vi "newest map.vi"() -> (1 "newest map":path[](array[path]))   [LabVIEW 2014]
panel:
  out "last mod":timestamp
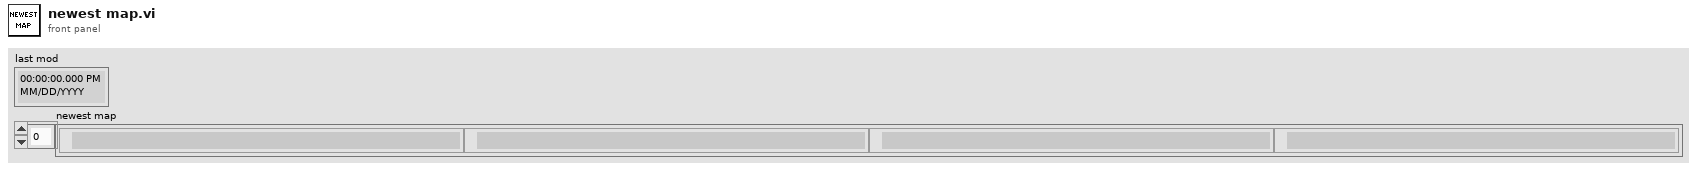
[diagram p1: front panel]
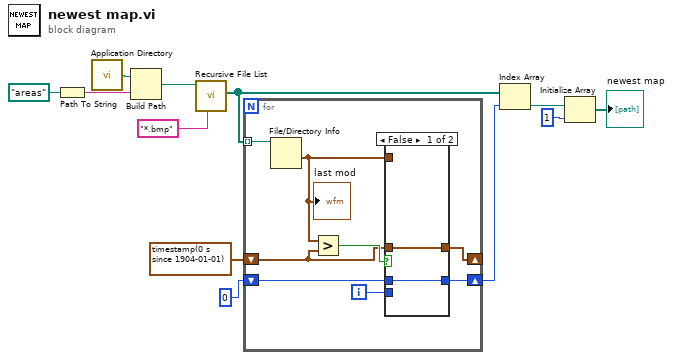
[diagram p0: block diagram]
diagram:
  n1 = Path To String(path=path "areas") -> (string=w2:string)
  n2 = call <vilib>:"Application Directory.vi"() -> ("Application Directory"=w4:path)
  n3 = Build Path(base path=w4, name or relative path=w2) -> (appended path=w1:path)
  n4 = call <vilib>:"Recursive File List.vi"("pattern"="*.bmp", "Folder Path"=w1) -> ("All Files in Dir"=w10:path[])  [unwired: 5 in, 4 out]
  n5 = for {
    tunnel: w10 -> [w20] mode=indexing
    shift-right: [w15] -> _
    shift-left: timestamp(0 s since 1904-01-01) ("last mod") -> [w14]
    shift-right: [w17] -> w9
    shift-left: 0 -> [w13]
    i -> [w18]
    n6 = File/Directory Info(path=w20) -> (last mod=w16:timestamp)  [unwired: 1 in, 6 out]
    "last mod" <- w16
    n7 = Greater?(x=w16, y=w14) -> (0:w19:bool)
    n8 = case shown="False" w19 {
      tunnel: w18 -> [_ w24]
      tunnel: [w21 w24] -> w17
      tunnel: w16 -> [_ w23]
      tunnel: [w22 w23] -> w15
      tunnel: w14 -> [w22 _]
      tunnel: w13 -> [w21 _]
      frame False {
      }
      frame True {
      }
    }
  }
  n9 = Index Array(array=w10, index=w9) -> (element=w6:path)
  n10 = Initialize Array(w6, 1 ("dimension size")) -> (→"newest map":path[])
